vi "Exit.vi"(8 "error in (no error)":errorcluster, 11 "Object ref in":T1) -> (0 "error out":errorcluster, 3 "Object ref out":T1)   [LabVIEW 2013, in "SLMControl.lvlib" / "SC-Main.lvclass"]
uses:
  SC-Main.lvclass
  Object-reference.ctl
  Deposition-actions.ctl
  Lasing-actions.ctl
  UI/Control-names.ctl
  SC-Main.lvclass/SC-Main.ctl
  Read UI.vi
  UI/Set-control-boolean.vi
  UI/SC-UI.lvclass
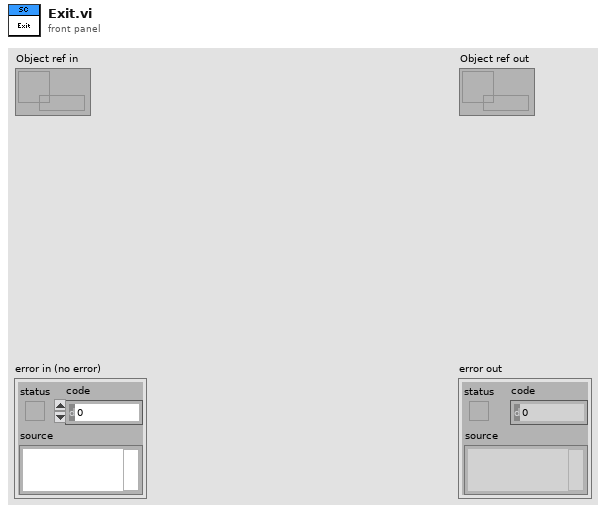
[diagram p1: front panel]
types:
  T1 = typedef "SLMControl.lvlib/SC-Main.lvclass/Object-reference.ctl" = refnum<data-value>
  T2 = typedef "SLMControl.lvlib/SC-UI.lvclass/Control-names.ctl" = enum16{"Com-in", "Com-out", "Help", "Status", "Load configuration", "Save configuration", "Load lasing files", "Load deposition files", "Clear", "Files", "Activate", "Execute", "Abort", "Options", "Current layer", "Current iteration", "Last elapsed time", "Deposition status", "Lasing job", "Status LEDs", "Exiting led", "Initialized led", "Files loaded led", "Activated led", "Executing led", "Deposition led", "Lasing job led", "Lasing led"}
  T3 = typedef "SLMControl.lvlib/SC-Main.lvclass/Lasing-actions.ctl" = enum16{"Idle", "Activate", "Load lasing file", "Launch lasing", "Wait for lasing end", "Signal iterate", "Signal abort", "Abort", "Reset", "Exit"}
  T4 = typedef "SLMControl.lvlib/SC-Main.lvclass/Deposition-actions.ctl" = enum16{"Idle", "Activate", "Load deposition", "Launch deposition", "Wait for deposition end", "Signal lasing", "Abort", "Reset", "Exit"}
  T5 = typedef "SLMControl.lvlib/SC-UI.lvclass/Panes-reference.ctl" = refnum<data-value>
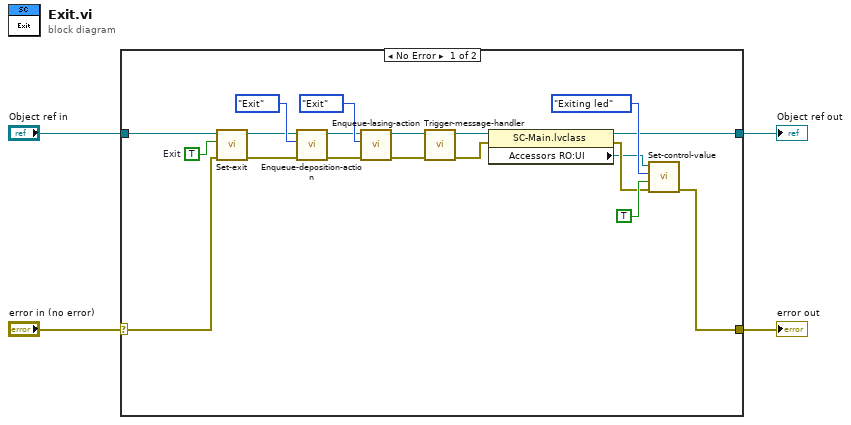
[diagram p0: block diagram]
diagram:
  n1 = case shown="No Error" "error in (no error)" {
    selector: "error in (no error)" -> [w21 w25]
    tunnel: [w5 w25] -> w3
    tunnel: [w6 w24] -> w1
    tunnel: "Object ref in" -> [w22 w24]
    frame No Error {
      w23 = TRUE  # Exit
      n2 = call "Set-exit.vi"("error in (no error)"=w21, "Exit?"=w23, "Object ref in"=w22) -> ("error out"=w15:errorcluster, "Object ref out"=w16:T1)  [unwired: 7 in]
      n3 = call "Enqueue-deposition-action.vi"("error in (no error)"=w15, "Action"=Deposition-actions."Exit" ("Execution action"), "State queue in"=w16) -> ("error out"=w17:errorcluster, "State queue out"=w18:T1)  [unwired: 6 in, 1 out]
      n4 = call "Enqueue-lasing-action.vi"("error in (no error)"=w17, "Action"=Lasing-actions."Exit" ("Execution action"), "State queue in"=w18) -> ("error out"=w10:errorcluster, "State queue out"=w14:T1)  [unwired: 6 in, 1 out]
      n5 = call "Trigger-message-handler.vi"("error in (no error)"=w10, "Object ref in"=w14) -> ("error out"=w9:errorcluster, "Object ref out"=w11:T1)  [unwired: 8 in]
      n6 = property class="SC-Main.lvclass"(reference=w11, error in=w9) -> (reference out=w6:T1, error out=w8:errorcluster, "Accessors RO:UI"=w7:T5)
      n7 = call-poly "Set-control-value.vi"("error in (no error)"=w8, "Value"=TRUE, "Control name"=Control-names."Exiting led", "Panes in"=w7) -> ("error out"=w5:errorcluster)  [unwired: 6 in, 1 out]
    }
    frame Error {
    }
  }
  "error out" <- w3
  "Object ref out" <- w1
